vi "显示测试结果-左上角.vi"(8 "显示坐标":cluster{dbl, "Numeric":dbl}[](array[cluster])=[{250.0, "Numeric"=430.0}], 9 "量测项目名称":string[](array[string]), 10 "存档信息":T1, 11 "引用句柄输入":T2) -> ()   [LabVIEW 2014]
uses:
  <vilib>/vision/Image Controls.llb/IMAQ Image.ctl
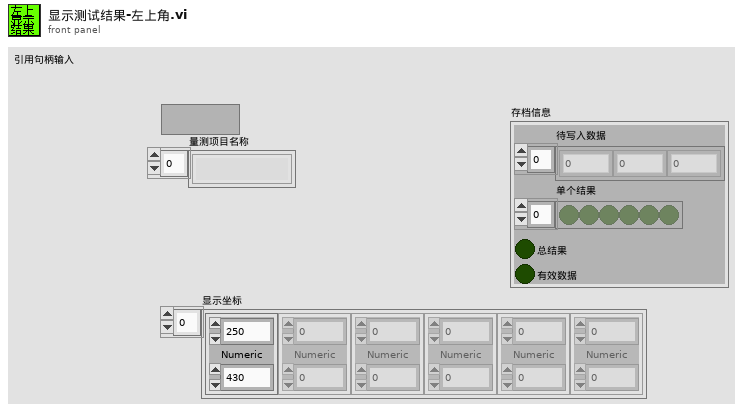
[diagram p1: front panel]
types:
  T1 = typedef "控件-存档数据和结果.ctl" = cluster{"待写入数据":dbl[], "单个结果":bool[], "总结果":bool, "有效数据":bool}
  T2 = typedef "IMAQ Image.ctl" = refnum<image>
  T3 = cluster{"Desired Font (Application)":enum16{"User-specified Font", "Application Font", "System Font", "Dialog Font"}, "[User-specified Font]":cluster{"Font Name":string, "Size":i16, "Strikeout?":bool, "Italic?":bool, "Underline?":bool, "Outline?":bool, "Shadow?":bool, "Bold?":bool, "Rotation Angle":dbl}, "Horizontal Alignment":i16, "Vertical Alignment":i16}
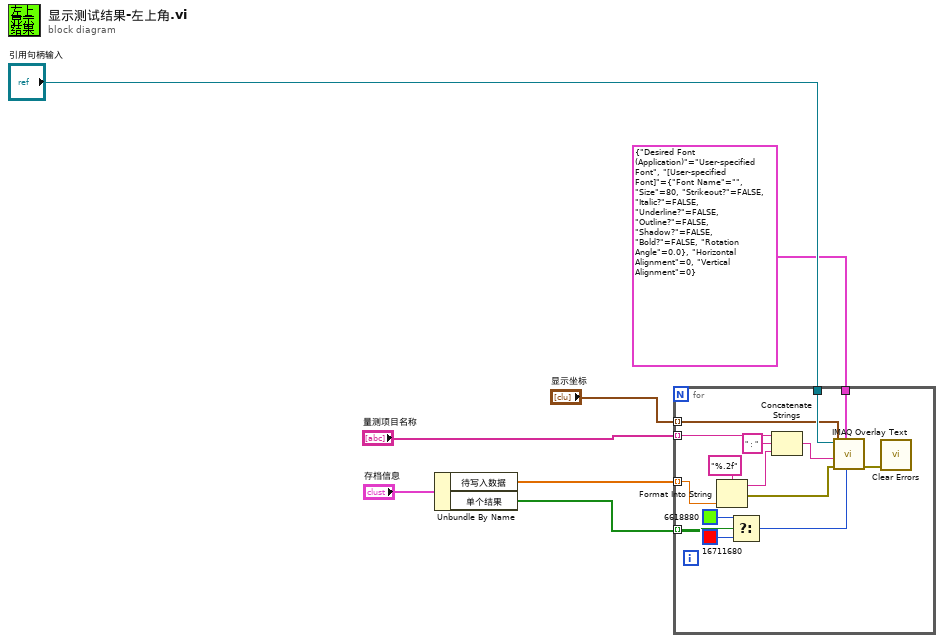
[diagram p0: block diagram]
diagram:
  n1 = Unbundle By Name("存档信息") -> ("待写入数据"=w3:dbl[], "单个结果"=w2:bool[])
  n2 = for {
    tunnel: "引用句柄输入" -> [w22]
    tunnel: w3 -> [w21] mode=indexing
    tunnel: "显示坐标" -> [w19] mode=indexing
    tunnel: w2 -> [w20] mode=indexing
    tunnel: T3 {"Desired Font (Application)"=enum."User-specified Font", "[User-specified Font]"={"Font Name"="", "Size"=80, "Strikeout?"=FALSE, "Italic?"=FALSE, "Underline?"=FALSE, "Outline?"=FALSE, "Shadow?"=FALSE, "Bold?"=FALSE, "Rotation Angle"=0.0}, "Horizontal Alignment"=0, "Vertical Alignment"=0} ("Font, Size & Style") -> [w18]
    tunnel: "量测项目名称" -> [w11] mode=indexing
    n3 = Format Into String(format string="%.2f" ("格式字符串"), w21) -> (resulting string=w9:string, error out=w13:errorcluster)  [unwired: 2 in]
    n4 = Select(t=u32 6618880 ("Text Color (black)"), s=w20, f=u32 16711680 ("Text Color (black)")) -> (s? t:f=w14:u32)
    n5 = Concatenate Strings(w11, "：" ("字符串"), w9) -> (w10:string)
    n6 = call "IMAQ Overlay Text"("Text Color (black)"=w14, "Font, Size & Style"=w18, "error in (no error)"=w13, "String"=w10, "Origin"=w19, "Image"=w22) -> ("error out"=w12:errorcluster)  [unwired: 4 in, 1 out]
    n7 = call <vilib>:"Clear Errors.vi"("error in (no error)"=w12) -> ()  [unwired: 5 in, 2 out]
  }
